vi "Parse_control_array_AMI.vi"(1 "Messreihe":i32) -> ()   [LabVIEW 2016]
uses:
  Global Variables/global.vi
  Global Variables/Data_Display_global.vi
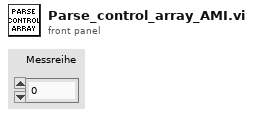
[diagram p1: front panel]
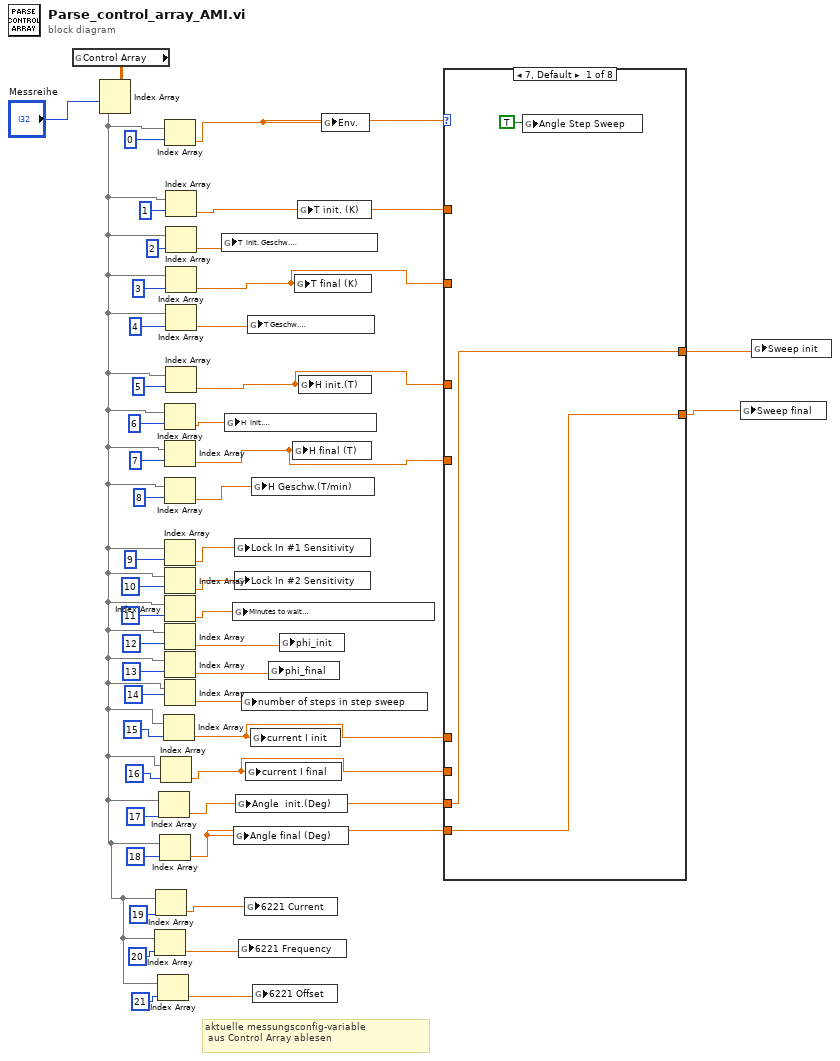
[diagram p0: block diagram]
diagram:
  # "aktuelle messungsconfig-variable\n aus Control Array ablesen"
  n1 = global read "global.vi" "Control Array"() -> (w49:dbl[][])
  n2 = Index Array(array=w49, index (row)="Messreihe") -> (element=w1:dbl[])  [unwired: 1 in]
  n3 = Index Array(array=w1, index=20) -> (element=w6:dbl)
  n4 = Index Array(array=w1, index=19) -> (element=w7:dbl)
  n5 = Index Array(array=w1, index=21) -> (element=w3:dbl)
  n6 = Index Array(array=w1, index=17) -> (element=w11:dbl)
  n7 = Index Array(array=w1, index=18) -> (element=w10:dbl)
  n8 = Index Array(array=w1, index=16) -> (element=w12:dbl)
  n9 = Index Array(array=w1, index=15) -> (element=w13:dbl)
  n10 = Index Array(array=w1, index=0) -> (element=w18:dbl)
  n11 = Index Array(array=w1, index=6) -> (element=w31:dbl)
  n12 = Index Array(array=w1, index=7) -> (element=w14:dbl)
  n13 = Index Array(array=w1, index=8) -> (element=w30:dbl)
  n14 = Index Array(array=w1, index=9) -> (element=w28:dbl)
  n15 = Index Array(array=w1, index=10) -> (element=w27:dbl)
  n16 = Index Array(array=w1, index=11) -> (element=w26:dbl)
  n17 = Index Array(array=w1, index=12) -> (element=w25:dbl)
  n18 = Index Array(array=w1, index=13) -> (element=w24:dbl)
  n19 = Index Array(array=w1, index=14) -> (element=w23:dbl)
  n20 = Index Array(array=w1, index=1) -> (element=w17:dbl)
  n21 = Index Array(array=w1, index=2) -> (element=w33:dbl)
  n22 = Index Array(array=w1, index=3) -> (element=w16:dbl)
  n23 = Index Array(array=w1, index=4) -> (element=w32:dbl)
  n24 = Index Array(array=w1, index=5) -> (element=w15:dbl)
  n25 = global write "global.vi" "T  init. Geschw. \n(K/min)"(w33) -> ()
  n26 = global write "global.vi" "H  init. \nGeschw.(T/min)"(w31) -> ()
  n27 = global write "global.vi" "Minutes to wait\nafter initialization"(w26) -> ()
  n28 = global write "global.vi" "Angle final (Deg)"(w10) -> ()
  n29 = global write "global.vi" "Lock In #1 Sensitivity"(w28) -> ()
  n30 = global write "global.vi" "Lock In #2 Sensitivity"(w27) -> ()
  n31 = global write "global.vi" "Angle  init.(Deg)"(w11) -> ()
  n32 = global write "global.vi" "6221 Frequency"(w6) -> ()
  n33 = global write "global.vi" "number of steps in step sweep"(w23) -> ()
  n34 = global write "global.vi" "6221 Current"(w7) -> ()
  n35 = global write "global.vi" "current I final"(w12) -> ()
  n36 = global write "global.vi" "T Geschw. \n(K/min)"(w32) -> ()
  n37 = global write "global.vi" "current I init"(w13) -> ()
  n38 = global write "global.vi" "H Geschw.(T/min)"(w30) -> ()
  n39 = global write "global.vi" "6221 Offset"(w3) -> ()
  n40 = global write "global.vi" "phi_final"(w24) -> ()
  n41 = global write "global.vi" "phi_init"(w25) -> ()
  n42 = global write "global.vi" "H final (T)"(w14) -> ()
  n43 = global write "global.vi" "T final (K)"(w16) -> ()
  n44 = global write "global.vi" "T init. (K)"(w17) -> ()
  n45 = global write "global.vi" "H init.(T)"(w15) -> ()
  n46 = global write "global.vi" "Env."(w18) -> ()
  n47 = case shown="7, Default" w18 {
    tunnel: w17 -> [_ _ w56 w58 _ _ w64 _]
    tunnel: w16 -> [_ _ w55 _ _ _ _ _]
    tunnel: w15 -> [_ w54 _ _ w60 _ w63 _]
    tunnel: w14 -> [_ w53 _ w57 w59 _ _ _]
    tunnel: w13 -> [_ _ _ _ _ w62 _ _]
    tunnel: w12 -> [_ _ _ _ _ w61 _ _]
    tunnel: w11 -> [w51 _ _ _ _ _ _ w66]
    tunnel: w10 -> [w50 _ _ _ _ _ _ w65]
    tunnel: [w51 w54 w56 w58 w60 w62 w64 w66] -> w9
    tunnel: [w50 w53 w55 w57 w59 w61 w63 w65] -> w8
    frame 7, Default {
      n48 = global write "Data_Display_global.vi" "Angle Step Sweep"(TRUE) -> ()
    }
    frame 1 {
    }
    frame 2 {
    }
    frame 3 {
    }
    frame 4 {
    }
    frame 5 {
    }
    frame 6 {
    }
    frame 8 {
    }
  }
  n49 = global write "global.vi" "Sweep final"(w8) -> ()
  n50 = global write "global.vi" "Sweep init"(w9) -> ()
